vi "Sweep States.vi"(8 "error in (no error)":errorcluster, 11 "Generator in":refnum<class "Generator.lvclass">) -> (0 "error out":errorcluster, 2 "Waveforms out":waveform(dbl)[](array[waveform]), 3 "Generator out":refnum<class "Generator.lvclass">)   [LabVIEW 2019, in "Generator.lvclass"]
uses:
  Generator.lvclass
  typedefs/Generator.Command--enum.ctl
  typedefs/Generator.Sweep State--enum.ctl
  Generator.lvclass/Generator.ctl
  typedefs/Generator.Sweep Status--enum.ctl
  Waveform.Attributes/Waveform.Attributes.lvlib
panel:
  out "new command?":bool
  out "iteration":i32
  out "state out":T1=enum."sweep"
  out "processed state":T1=enum."sweep"
  out "state in":T1=enum."sweep"
  out "command":T2=enum."stop sweep"
  out "Waveform Chart":dbl(graph)
  out "sweep duration":dbl
  out "start sweep time":timestamp
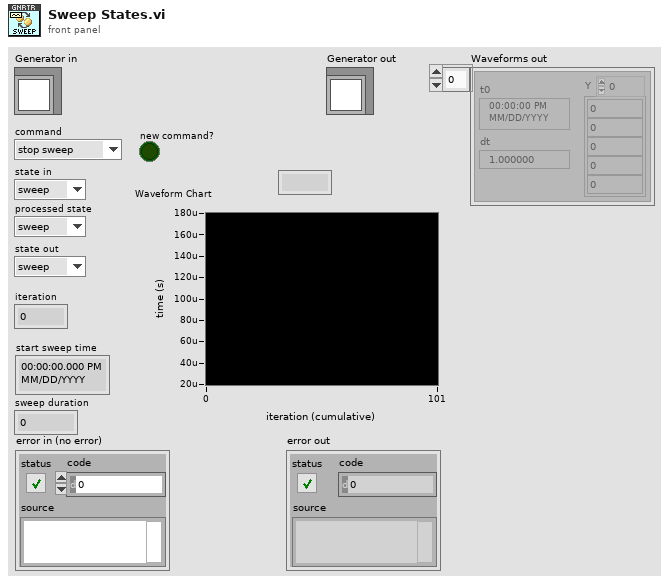
[diagram p1: front panel]
types:
  T1 = typedef "Generator.lvclass/Generator.Sweep State--enum.ctl" = enum16{"idle", "initialize", "wait", "sweep", "stop"}
  T2 = typedef "Generator.lvclass/Generator.Command--enum.ctl" = enum16{"start", "stop", "start sweep", "stop sweep"}
  T3 = typedef "Generator.lvclass/Generator.Sweep Status--enum.ctl" = enum16{"idle", "initializing", "waiting", "sweeping", "stopping"}
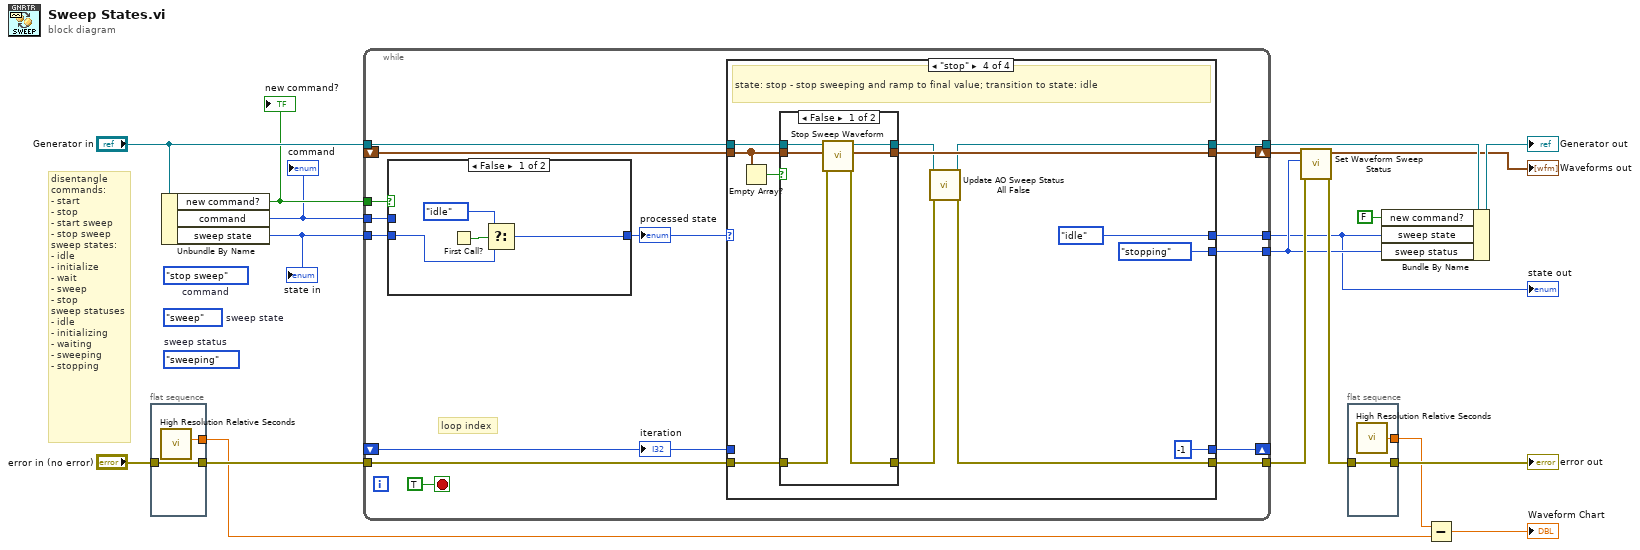
[diagram p0: block diagram]
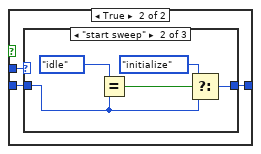
[diagram p2: hidden frame]
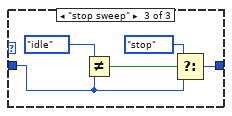
[diagram p4: hidden frame]
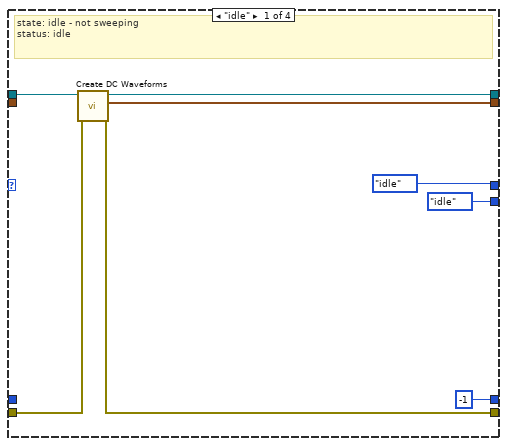
[diagram p5: hidden frame]
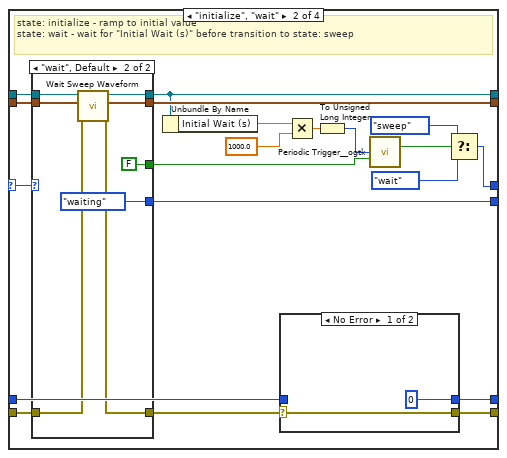
[diagram p6: hidden frame]
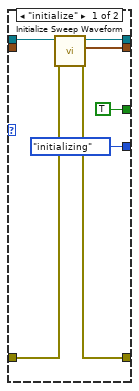
[diagram p7: hidden frame]
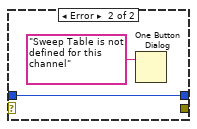
[diagram p8: hidden frame]
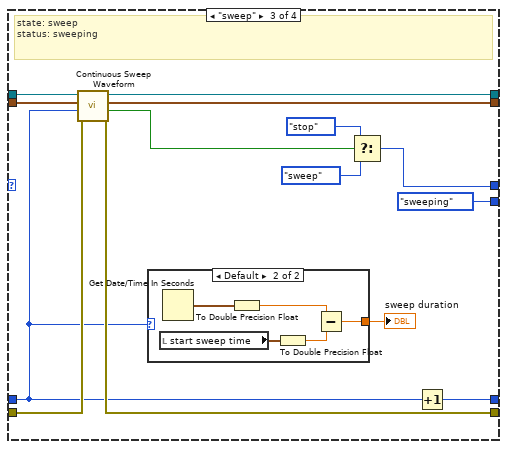
[diagram p9: hidden frame]
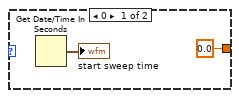
[diagram p10: hidden frame]
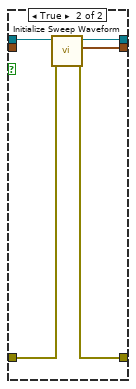
[diagram p11: hidden frame]
diagram:
  (unwired) Generator.Command--enum."stop sweep"  # command
  (unwired) Generator.Sweep_State--enum."sweep"  # sweep state
  (unwired) Generator.Sweep_Status--enum."sweeping"  # sweep status
  # "disentangle\ncommands:\n- start\n- stop\n- start sweep\n- stop sweep\nsweep states:\n- idle\n- initialize\n- wait\n- sweep\n- stop\nsweep statuses\n- idle\n- initializing\n- waiting\n- sweeping\n- stopping"
  n1 = flat-sequence {
    tunnel: "error in (no error)" -> [w21]
    tunnel: [w21] -> w18
    tunnel: [w20] -> w8
    frame #0 {
      n2 = call <vilib>:"High Resolution Relative Seconds.vi"() -> ("relative seconds"=w20:dbl)
    }
  }
  n3 = Unbundle By Name("Generator in") -> ("new command?"=w4:bool, "command"=w3:T2, "sweep state"=w5:T1)
  "command" <- w3
  "state in" <- w5
  "new command?" <- w4
  n4 = while {
    shift-right: [w36] -> _
    shift-left: _ -> [w31]
    tunnel: [w34] -> w10
    tunnel: "Generator in" -> [w28]
    tunnel: w18 -> [w33]
    tunnel: [w32] -> w14
    shift-right: [w30] -> w15
    shift-left: _ -> [w29]
    tunnel: [w26] -> w6
    tunnel: w5 -> [w25]
    tunnel: [w27] -> w2
    tunnel: w4 -> [w24]
    tunnel: w3 -> [w23]
    stop <- TRUE stop-if-true
    # "loop index"
    n5 = case shown="False" w24 {
      tunnel: w25 -> [w37 w41]
      tunnel: [w38 w42] -> w22
      tunnel: w23 -> [_ w43]
      frame False {
        n6 = First Call?() -> (First Call?: T/F=w40:bool)
        n7 = Select(t=Generator.Sweep_State--enum."idle", s=w40, f=w37) -> (s? t:f=w38:T1)
      }
      frame True {
        n8 = case shown="\"start sweep\"" w43 {
          tunnel: [w44 w45 w50] -> w42
          tunnel: w41 -> [w44 w46 w51]
          frame Default {
          }
          frame "start sweep" {
            n9 = Equal?(x=Generator.Sweep_State--enum."idle" ("sweep state"), y=w46) -> (x = y?=w49:bool)
            n10 = Select(t=Generator.Sweep_State--enum."initialize" ("sweep state"), s=w49, f=w46) -> (s? t:f=w45:T1)
          }
          frame "stop sweep" {
            n11 = Not Equal?(x=Generator.Sweep_State--enum."idle" ("sweep state"), y=w51) -> (x != y?=w54:bool)
            n12 = Select(t=Generator.Sweep_State--enum."stop" ("sweep state"), s=w54, f=w51) -> (s? t:f=w50:T1)
          }
        }
      }
    }
    "processed state" <- w22
    n13 = case shown="\"stop\"" w22 {
      selector: w22 -> [_ w67 _ _]
      tunnel: [-1 w82 w115 -1] -> w36
      tunnel: w31 -> [_ w77 w110 _]
      tunnel: [w58 w71 w107 w126] -> w34
      tunnel: w33 -> [w61 w81 w112 w134]
      tunnel: [w60 w78 w111 w124] -> w32
      tunnel: [w59 w80 w109 w127] -> w30
      tunnel: w28 -> [w57 w74 w114 w133]
      tunnel: w29 -> [_ w66 w113 w131]
      tunnel: [Generator.Sweep_State--enum."idle" ("sweep state in 2") w73 w104 Generator.Sweep_State--enum."idle" ("sweep state in 2")] -> w27
      tunnel: [Generator.Sweep_Status--enum."idle" ("sweep status") w63 Generator.Sweep_Status--enum."sweeping" ("sweep status") Generator.Sweep_Status--enum."stopping" ("sweep status")] -> w26
      frame "idle" {
        # "state: idle - not sweeping\nstatus: idle"
        n14 = call "Create DC Waveforms.vi"("error in (no error)"=w61, "Generator in"=w57) -> ("Error out"=w60:errorcluster, "Waveforms out"=w59:waveform(dbl)[], "Generator out"=w58:refnum<class "Generator.lvclass">)  [unwired: 7 in]
      }
      frame "initialize", "wait" {
        # "state: initialize - ramp to initial value\nstate: wait - wait for \"Initial Wait (s)\" before transition to state: sweep"
        n15 = case shown="\"wait\", Default" w67 {
          tunnel: w81 -> [w89 w91]
          tunnel: [w88 w96] -> w80
          tunnel: [w87 w92] -> w79
          tunnel: w74 -> [w86 w94]
          tunnel: [w85 w95] -> w71
          tunnel: [TRUE ("reset") FALSE ("reset")] -> w69
          tunnel: w66 -> [_ w93]
          tunnel: [Generator.Sweep_Status--enum."initializing" ("sweep status") Generator.Sweep_Status--enum."waiting" ("sweep status")] -> w63
          frame "initialize" {
            n16 = call "Initialize Sweep Waveform.vi"("error in (no error)"=w89, "Generator in"=w86) -> ("error out"=w87:errorcluster, "Waveforms"=w88:waveform(dbl)[], "Generator out"=w85:refnum<class "Generator.lvclass">)  [unwired: 7 in]
          }
          frame "wait", Default {
            n17 = call "Wait Sweep Waveform.vi"("error in (no error)"=w91, "Waveforms in"=w93, "Generator in"=w94) -> ("error out"=w92:errorcluster, "Waveforms out"=w96:waveform(dbl)[], "Generator out"=w95:refnum<class "Generator.lvclass">)  [unwired: 6 in]
          }
        }
        n18 = Unbundle By Name(w71) -> ("Initial Wait (s)"=w76:dbl)
        n19 = case shown="No Error" w79 {
          selector: w79 -> [w98 _]
          tunnel: [0 w101] -> w82
          tunnel: w77 -> [_ w101]
          tunnel: [w98 _] -> w78
          frame No Error {
          }
          frame Error {
            n20 = One Button Dialog(message="Sweep Table is not defined for this channel") -> ()  [unwired: 1 in, 1 out]
          }
        }
        n21 = Multiply(x=w76, y=1000.0) -> (x*y=w75:dbl)
        n22 = To Unsigned Long Integer(number=w75) -> (unsigned 32bit integer=w70:u32)
        n23 = call <userlib>:"Periodic Trigger__ogtk.vi"("time (ms)"=w70, "reset"=w69) -> ("Triggered"=w72:bool)  [unwired: 11 in, 2 out]
        n24 = Select(t=Generator.Sweep_State--enum."sweep" ("sweep state"), s=w72, f=Generator.Sweep_State--enum."wait" ("sweep state")) -> (s? t:f=w73:T1)
      }
      frame "sweep" {
        # "state: sweep\nstatus: sweeping"
        n25 = call "Continuous Sweep Waveform.vi"("error in (no error)"=w112, "Sweep Index"=w110, "Waveforms in"=w113, "Generator in"=w114) -> ("error out"=w111:errorcluster, "finished?"=w106:bool, "Waveforms out"=w109:waveform(dbl)[], "Generator in"=w107:refnum<class "Generator.lvclass">)  [unwired: 4 in]
        n26 = case shown="Default" w110 {
          tunnel: [0.0 w118] -> w102
          frame 0 {
            n27 = Get Date/Time In Seconds() -> (seconds since 1Jan1904=→"start sweep time":timestamp)
          }
          frame Default {
            n28 = local read "start sweep time"() -> (w122:timestamp)
            n29 = Get Date/Time In Seconds() -> (seconds since 1Jan1904=w121:timestamp)
            n30 = To Double Precision Float(number=w121) -> (double precision float=w120:dbl)
            n31 = To Double Precision Float(number=w122) -> (double precision float=w119:dbl)
            n32 = Subtract(x=w120, y=w119) -> (x-y=w118:dbl)
          }
        }
        "sweep duration" <- w102
        n33 = Select(t=Generator.Sweep_State--enum."stop" ("sweep state"), s=w106, f=Generator.Sweep_State--enum."sweep" ("sweep state")) -> (s? t:f=w104:T1)
        n34 = Increment(x=w110) -> (x+1=w115:i32)
      }
      frame "stop" {
        # "state: stop - stop sweeping and ramp to final value; transition to state: idle"
        n35 = Empty Array?(array=w131) -> (empty?=w132:bool)
        n36 = case shown="False" w132 {
          tunnel: w134 -> [w140 w143]
          tunnel: w133 -> [w139 w145]
          tunnel: [w138 w144] -> w123
          tunnel: [w137 w142] -> w125
          tunnel: [w136 w141] -> w127
          tunnel: w131 -> [w135 _]
          frame False {
            n37 = call "Stop Sweep Waveform.vi"("error in (no error)"=w140, "Waveforms in"=w135, "Generator in"=w139) -> ("error out"=w137:errorcluster, "Waveforms out"=w136:waveform(dbl)[], "Generator out"=w138:refnum<class "Generator.lvclass">)  [unwired: 6 in]
          }
          frame True {
            n38 = call "Initialize Sweep Waveform.vi"("error in (no error)"=w143, "Generator in"=w145) -> ("error out"=w142:errorcluster, "Waveforms"=w141:waveform(dbl)[], "Generator out"=w144:refnum<class "Generator.lvclass">)  [unwired: 7 in]
          }
        }
        n39 = call "Update AO Sweep Status All False.vi"("error in (no error)"=w125, "Generator in"=w123) -> ("error out"=w124:errorcluster, "Generator out"=w126:refnum<class "Generator.lvclass">)  [unwired: 8 in]
      }
    }
    "iteration" <- w31
  }
  "state out" <- w2
  n40 = call "Set Waveform Sweep Status.vi"("error in (no error)"=w14, "sweep status"=w6, "Waveforms in"=w15) -> ("error out"=w13:errorcluster, "Waveforms out"=→"Waveforms out":waveform(dbl)[])  [unwired: 7 in]
  n41 = flat-sequence {
    tunnel: w13 -> [w147]
    tunnel: [w147] -> w17
    tunnel: [w146] -> w16
    frame #0 {
      n42 = call <vilib>:"High Resolution Relative Seconds.vi"() -> ("relative seconds"=w146:dbl)
    }
  }
  n43 = Bundle By Name(cluster=w10, "new command?"=FALSE, "sweep state"=w2, "sweep status"=w6) -> (→"Generator out":refnum<class "Generator.lvclass">)
  n44 = Subtract(x=w16, y=w8) -> (x-y=→"Waveform Chart":dbl)
  "error out" <- w17
